vi "Error站_GetData.vi"(0 "ref in":T4, 11 "error in":errorcluster) -> (3 "Flag out":T3, 4 "ref out":T4, 6 "Ready":bool, 8 "Mode":T2, 10 "Function":T1, 14 "Data out":T5, 15 "error out":errorcluster)   [LabVIEW 2015]
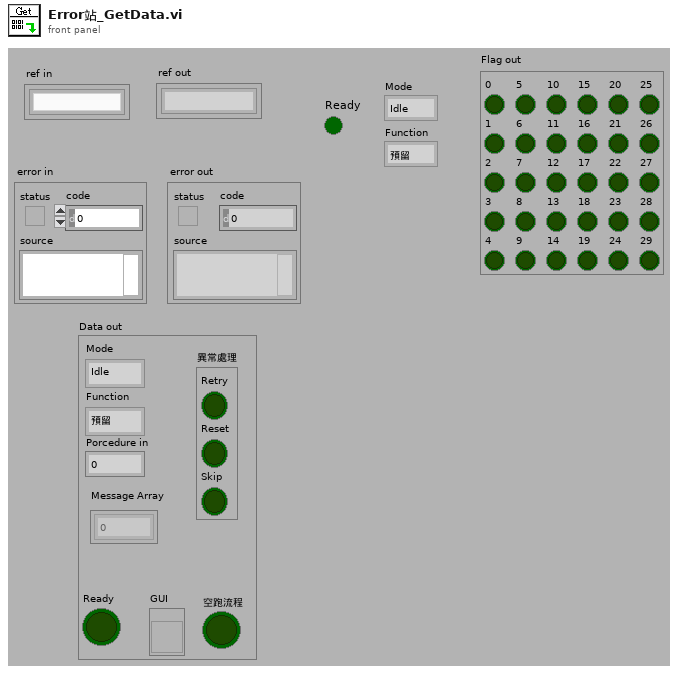
[diagram p1: front panel]
types:
  T1 = typedef "Error站_Function.ctl" = enum8{"預留"}
  T2 = typedef "Error站_Mode.ctl" = enum8{"Idle", "Run", "Pause", "Err"}
  T3 = typedef "Error站_Flag.ctl" = cluster{"0":bool, "1":bool, "2":bool, "3":bool, "4":bool, "5":bool, "6":bool, "7":bool, "8":bool, "9":bool, "10":bool, "11":bool, "12":bool, "13":bool, "14":bool, "15":bool, "16":bool, "17":bool, "18":bool, "19":bool, "20":bool, "21":bool, "22":bool, "23":bool, "24":bool, "25":bool, "26":bool, "27":bool, "28":bool, "29":bool}
  T4 = typedef "Error站_ref.ctl" = refnum<k1>
  T5 = typedef "Error站_Data.ctl" = cluster{"GUI":refnum<vi>, "Ready":bool, "Mode":T2, "Function":T1, "Porcedure in":u8, "空跑流程":bool, "異常處理":cluster{"Retry":bool, "Reset":bool, "Skip":bool}, "Message Array":i32[]}
  T6 = enum16{"OpenReference", "CloseReference", "Get Data", "Set Data", "Set Flag"}
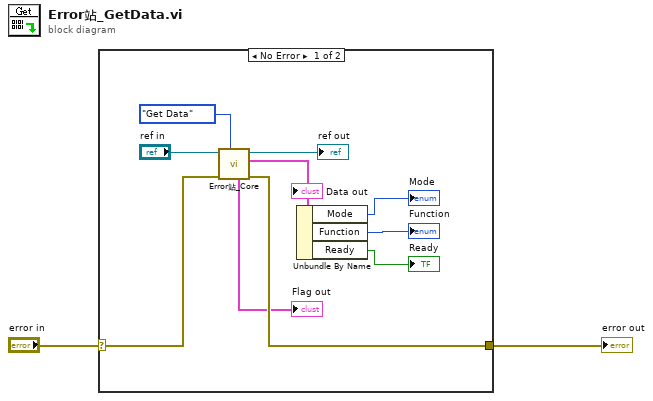
[diagram p0: block diagram]
diagram:
  n1 = case shown="No Error" "error in" {
    selector: "error in" -> [w12 w13]
    tunnel: [w11 w13] -> w1
    frame No Error {
      n2 = call "Error站_Core.vi"("Function"=T6."Get Data", "error in"=w12, "ref in"="ref in") -> ("error out"=w11:errorcluster, "Data out"=w10:T5, "ref out"=→"ref out":T4, "Flag out"=→"Flag out":T3)  [unwired: 5 in]
      "Data out" <- w10
      n3 = Unbundle By Name(w10) -> ("Mode"=→"Mode":T2, "Function"=→"Function":T1, "Ready"=→"Ready":bool)
    }
    frame Error {
    }
  }
  "error out" <- w1
